vi "LedMain.vi"(9 "Serial Port":T1, 10 "Mode":enum16{"Open", "Run"}(ring)) -> ()   [LabVIEW 2016]
uses:
  <vilib>/Rock Robotics/WPI/SerialPort/WPI_SerialPort.ctl
  LedStates.ctl
  <vilib>/Rock Robotics/WPI/DriverStation/WPI_DriverStationAllianceInfo.ctl
  <vilib>/Rock Robotics/Network Tables/NT Read Boolean.vi
  <vilib>/Rock Robotics/Network Tables/NT Read Number.vi
panel:
  out "Error Out":errorcluster
  in  "Error In":errorcluster
  # "2017 LED Main Control VI\nFRC Team 34"
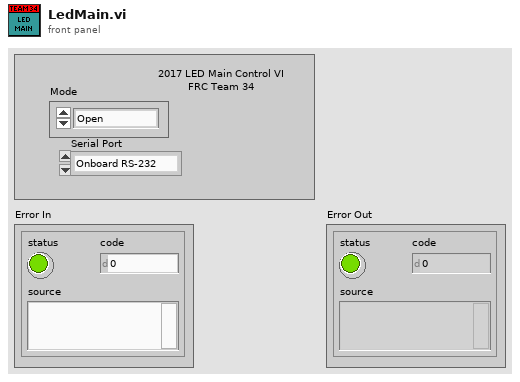
[diagram p1: front panel]
types:
  T1 = typedef "WPI_SerialPort.ctl" = enum16{"Onboard RS-232", "MXP TTL", "USB 1", "USB 2"}
  T2 = typedef "LedStates.ctl" = enum16{"Alliance", "Demo", "Police", "Train", "Climb", "Target Acquisition"}
  T3 = typedef "WPI_DriverStationAllianceInfo.ctl" = enum16{"Red", "Blue", "Invalid"}
  T4 = typedef "WPI_SerialPortRef.ctl" = cluster{"DevStatus":errorcluster, "Serial Port Name":refnum<visa-resource-name>}
  T5 = typedef "WPI_SwitchDevRef.ctl" = cluster{"DevStatus":errorcluster, "DIO Channel":T6, "CntIndex":T7, "Normally Closed":bool}
  T6 = typedef "FPGA_DIOChannel.ctl" = enum8{"DIO 0", "DIO 1", "DIO 2", "DIO 3", "DIO 4", "DIO 5", "DIO 6", "DIO 7", "DIO 8", "DIO 9", "DIO MXP 0", "DIO MXP 1", "DIO MXP 2", "DIO MXP 3", "DIO MXP 4", "DIO MXP 5", "DIO MXP 6", "DIO MXP 7", "DIO MXP 8", "DIO MXP 9", "DIO MXP 10", "DIO MXP 11", "DIO MXP 12", "DIO MXP 13", "DIO MXP 14", "DIO MXP 15", "SPI Port CS1", "SPI Port CS2", "SPI Port CS3", "SPI Port MISO", "SPI Port MOSI", "Invalid"}
  T7 = typedef "FPGA_CounterCtrSystemIndex.ctl" = enum8{"Ctr 0", "Ctr 1", "Ctr 2", "Ctr 3", "Ctr 4", "Ctr 5", "Ctr 6", "Ctr 7", "Invalid"}
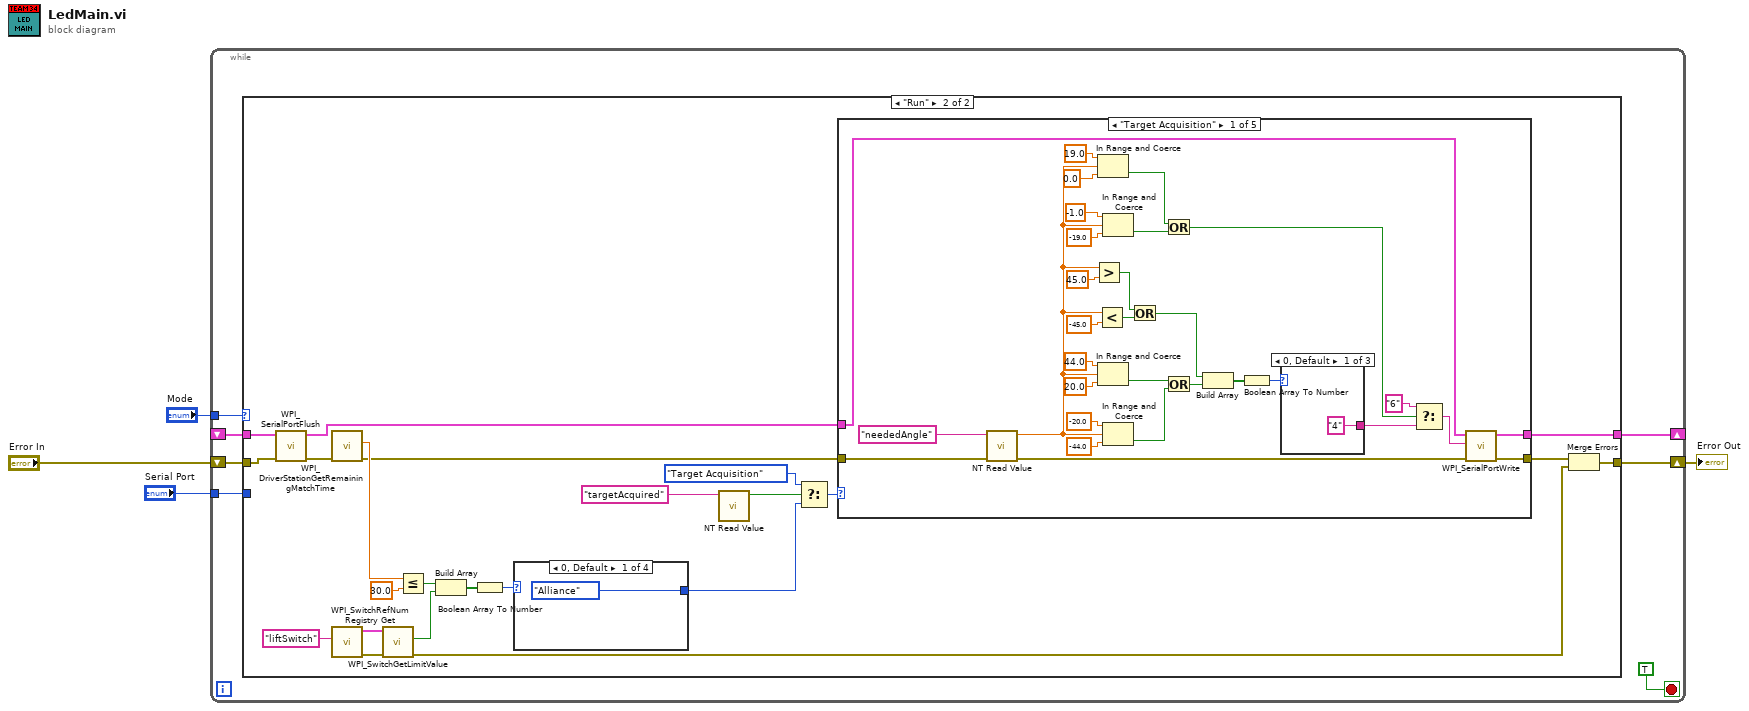
[diagram p0: block diagram]
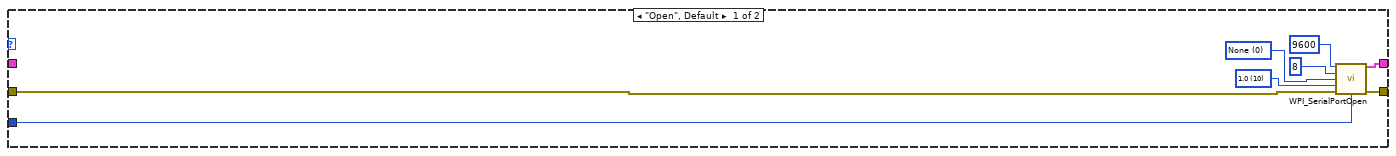
[diagram p2: hidden frame]
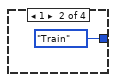
[diagram p3: hidden frame]
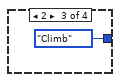
[diagram p4: hidden frame]
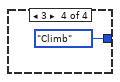
[diagram p5: hidden frame]
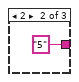
[diagram p6: hidden frame]
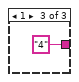
[diagram p7: hidden frame]
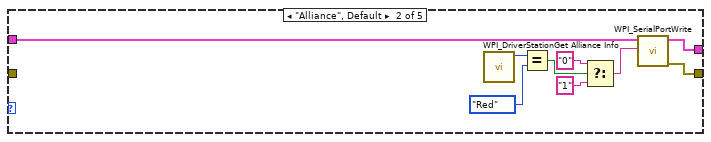
[diagram p8: hidden frame]
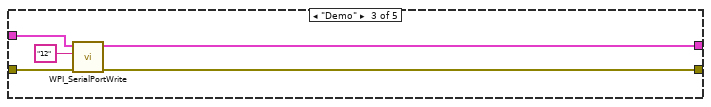
[diagram p9: hidden frame]
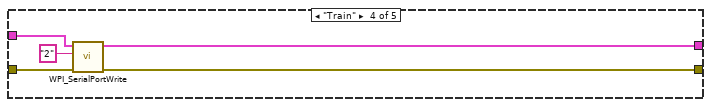
[diagram p10: hidden frame]
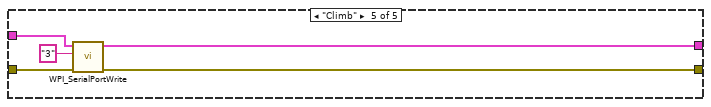
[diagram p11: hidden frame]
diagram:
  n1 = while {
    tunnel: "Mode" -> [w11]
    shift-right: [w9] -> w1
    shift-left: "Error In" -> [w8]
    shift-right: [w7] -> _
    shift-left: _ -> [w5]
    tunnel: "Serial Port" -> [w6]
    stop <- TRUE stop-if-true
    n2 = case shown="\"Run\"" w11 {
      tunnel: w8 -> [w15 w41]
      tunnel: [w14 w27] -> w9
      tunnel: [w13 w39] -> w7
      tunnel: w6 -> [w12 _]
      tunnel: w5 -> [_ w42]
      frame "Open", Default {
        w16 = u16 10 items=["1.0"=10, "1.5"=15, "2.0"=20] ("Stop Bits")
        w17 = u16 0 items=["None", "Odd", "Even", "Mark", "Space"] ("Parity")
        n3 = call <vilib>:"WPI_SerialPortOpen.vi"("Baud Rate"=u32 9600, "Data Bits"=u16 8, "Parity"=w17, "Stop Bits"=w16, "error in (no error)"=w15, "Serial Port"=w12) -> ("SerialPortRef"=w13:T4, "error out"=w14:errorcluster)  [unwired: 8 in]
      }
      frame "Run" {
        n4 = call <vilib>:"WPI_SerialPortFlush.vi"("error in (no error)"=w41, "SerialPortRef"=w42) -> ("error out"=w37:errorcluster, "SerialPortRef"=w40:T4)  [unwired: 8 in]
        n5 = call <vilib>:"WPI_DriverStationGetRemainingMatchTime.vi"("error in (no error)"=w37) -> ("error out"=w36:errorcluster, "Match Time(s)"=w38:sgl)  [unwired: 9 in]
        n6 = call <vilib>:"WPI_SwitchRefNum Registry Get.vi"("refnum name"="liftSwitch") -> ("error out"=w29:errorcluster, "SwitchDevRef"=w30:T5)  [unwired: 9 in]
        n7 = call <vilib>:"WPI_SwitchGetLimitValue.vi"("error in (no error)"=w29, "SwitchDevRef"=w30) -> ("error out"=w25:errorcluster, "Switch Pressed"=w26:bool)  [unwired: 7 in, 1 out]
        n8 = Less Or Equal?(x=w38, y=sgl 30.0) -> (x <= y?=w34:bool)
        n9 = Build Array(w34, w26) -> (w33:bool[])
        n10 = Boolean Array To Number(Boolean array=w33) -> (number=w32:u32)
        n11 = case shown="0, Default" w32 {
          tunnel: [LedStates."Alliance" LedStates."Train" LedStates."Climb" LedStates."Climb"] -> w21
          frame 0, Default {
          }
          frame 1 {
          }
          frame 2 {
          }
          frame 3 {
          }
        }
        n12 = call-poly <vilib>:"NT Read Value.vi"("Name"="targetAcquired") -> ("Boolean"=w23:bool)  [unwired: 9 in, 1 out]
        n13 = Select(t=LedStates."Target Acquisition", s=w23, f=w21) -> (s? t:f=w20:T2)
        n14 = case shown="\"Target Acquisition\"" w20 {
          tunnel: w40 -> [w74 w89 w91 w99 w101]
          tunnel: [w77 w88 w94 w97 w103] -> w28
          tunnel: [w76 w87 w93 w98 w102] -> w39
          tunnel: w36 -> [w75 _ w92 w96 w104]
          frame "Target Acquisition" {
            n15 = call-poly <vilib>:"NT Read Value.vi"("error in"=w75, "Name"="neededAngle") -> ("error out"=w47:errorcluster, "Numeric"=w52:dbl)  [unwired: 8 in]
            n16 = Greater?(x=w52, y=45.0) -> (0:w72:bool)
            n17 = Less?(x=w52, y=-45.0) -> (x < y?=w71:bool)
            n18 = In Range and Coerce(upper limit=19.0, x=w52, lower limit=0.0) -> (In Range?=w54:bool)  [unwired: 1 out]
            n19 = In Range and Coerce(upper limit=44.0, x=w52, lower limit=20.0) -> (In Range?=w63:bool)  [unwired: 1 out]
            n20 = In Range and Coerce(upper limit=-1.0, x=w52, lower limit=-19.0) -> (In Range?=w53:bool)  [unwired: 1 out]
            n21 = In Range and Coerce(upper limit=-20.0, x=w52, lower limit=-44.0) -> (In Range?=w62:bool)  [unwired: 1 out]
            n22 = Or(x=w72, y=w71) -> (x .or. y?=w73:bool)
            n23 = Or(x=w54, y=w53) -> (x .or. y?=w56:bool)
            n24 = Or(x=w63, y=w62) -> (x .or. y?=w61:bool)
            n25 = Build Array(w73, w61) -> (w60:bool[])
            n26 = Boolean Array To Number(Boolean array=w60) -> (number=w59:u32)
            n27 = case shown="0, Default" w59 {
              tunnel: ["4" "5" "4"] -> w57
              frame 0, Default {
              }
              frame 2 {
              }
              frame 1 {
              }
            }
            n28 = Select(t="6", s=w56, f=w57) -> (s? t:f=w58:string)
            n29 = call <vilib>:"WPI_SerialPortWrite.vi"("error in (no error)"=w47, "Buffer"=w58, "SerialPortRef"=w74) -> ("error out"=w77:errorcluster, "SerialPortRef"=w76:T4)  [unwired: 6 in, 1 out]
          }
          frame "Alliance", Default {
            n30 = call <vilib>:"WPI_DriverStationGet Alliance Info.vi"() -> ("Alliance"=w86:T3)  [unwired: 10 in, 1 out]
            n31 = Equal?(x=w86, y=WPI_DriverStationAllianceInfo."Red" ("Alliance")) -> (x = y?=w84:bool)
            n32 = Select(t="0", s=w84, f="1") -> (s? t:f=w81:string)
            n33 = call <vilib>:"WPI_SerialPortWrite.vi"("Buffer"=w81, "SerialPortRef"=w89) -> ("error out"=w88:errorcluster, "SerialPortRef"=w87:T4)  [unwired: 7 in, 1 out]
          }
          frame "Demo" {
            n34 = call <vilib>:"WPI_SerialPortWrite.vi"("error in (no error)"=w92, "Buffer"="12", "SerialPortRef"=w91) -> ("error out"=w94:errorcluster, "SerialPortRef"=w93:T4)  [unwired: 6 in, 1 out]
          }
          frame "Train" {
            n35 = call <vilib>:"WPI_SerialPortWrite.vi"("error in (no error)"=w96, "Buffer"="2", "SerialPortRef"=w99) -> ("error out"=w97:errorcluster, "SerialPortRef"=w98:T4)  [unwired: 6 in, 1 out]
          }
          frame "Climb" {
            n36 = call <vilib>:"WPI_SerialPortWrite.vi"("error in (no error)"=w104, "Buffer"="3", "SerialPortRef"=w101) -> ("error out"=w103:errorcluster, "SerialPortRef"=w102:T4)  [unwired: 6 in, 1 out]
          }
        }
        n37 = Merge Errors(w28, w25) -> (w27:errorcluster)
      }
    }
  }
  "Error Out" <- w1
